vi "Drive Controller.vi"(8 "error in":errorcluster) -> ()   [LabVIEW 2020]
doc: "This VI executes continuously carrying out the current operation and responding to updates or new operation requests. It will often contain the timing or control code that is difficult to place directly in TeleOp. This VI generally opens all sensors and motors and isolates the rest of the robot code from knowing implementation details of how the operations are carried out."
uses:
  <vilib>/Rock Robotics/WPI/Framework/Completion Status.ctl
  Drive Setpoints.ctl
  Drive Operations.ctl
  <vilib>/Rock Robotics/WPI/SafetyOutput/WPI_SafetyOutputConfigMenu.ctl
  <vilib>/Rock Robotics/WPI/RobotDrive/WPI_RobotDriveOpen2MotorWithExistingMotors.vi
  <vilib>/Rock Robotics/Network Tables/NT Write Numeric Array.vi
panel:
  in  "Interactive Values":T1
  in  "Buttons":cluster{"Execute Cmd":bool, "Abort Cmd":bool}
  out "Command Timing":cluster{"Start Time (ms)":u32, "Iterations":i32}
  out "Status":T3
  out "Setpoints":T4(graph)
  out "Current\nCmd":string
  # "Tip: The graph shows the motor setpoints. It may also be helpful to observe inputs and sensor values.\nYou may also want to display tuning or debugging controls."
  # "Interactive Command: You may fill in the settings for a command\nand schedule it with the Execute button. You can observe and abort\nany command while fine tuning the code for the controller."
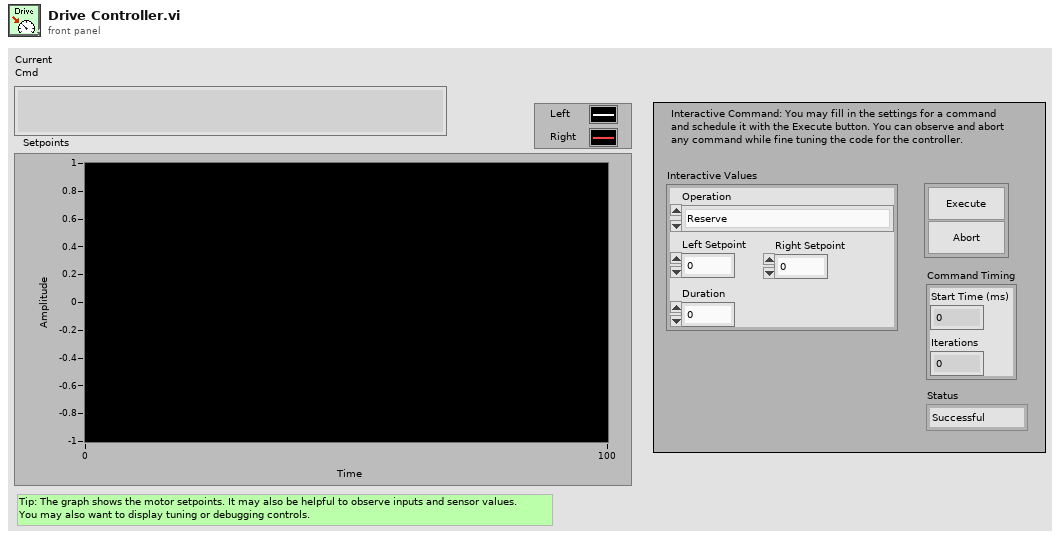
[diagram p1: front panel]
types:
  T1 = typedef "Drive Setpoints.ctl" = cluster{"Operation":T2, "Left Setpoint":dbl, "Right Setpoint":dbl, "Duration":dbl}
  T2 = typedef "Drive Operations.ctl" = enum16{"Reserve", "Read Current", "Immediate", "Drive for Time", "Drive for Distance"}
  T3 = typedef "Completion Status.ctl" = enum16{"Successful", "Aborted", "Incomplete"}
  T4 = cluster{"Left Setpoint":dbl, "Right Setpoint":dbl}
  T5 = typedef "WPI_SafetyOutputConfigMenu.ctl" = enum16{"Enable", "Disable"}
  T6 = typedef "WPI_MotorControlDeviceRef.ctl" = cluster{"DeviceStatus":errorcluster, "Type":T7, "PWM":cluster{"PWM Channel":T8, "DeadBand":T9}, "CAN":cluster{"Device Number":u8, "SetOutput VI Ref":variant, "GetOutput VI Ref":variant, "Enable VI Ref":variant, "Disable VI Ref":variant, "Data":variant}, "Invert":bool, "DIO PWM":cluster{"PWM \"Enable\" Channel":T8, "DIOChannel":T10, "PWM Rate":dbl}}
  T7 = typedef "WPI_MotorControlType.ctl" = enum16{"PWM", "CAN", "DIO PWM"}
  T8 = typedef "FPGA_DIOPWMChannel.ctl" = enum8{"PWM 0", "PWM 1", "PWM 2", "PWM 3", "PWM 4", "PWM 5", "PWM 6", "PWM 7", "PWM 8", "PWM 9", "PWM MXP 0", "PWM MXP 1", "PWM MXP 2", "PWM MXP 3", "PWM MXP 4", "PWM MXP 5", "PWM MXP 6", "PWM MXP 7", "PWM MXP 8", "PWM MXP 9", "Invalid"}
  T9 = typedef "WPI_PWMDeadband.ctl" = cluster{"Name":string, "maxPositivePwm":i32, "minPositivePwm":i32, "centerPwm":i32, "maxNegativePwm":i32, "minNegativePwm":i32, "angularRange":u16}
  T10 = typedef "FPGA_DIOChannel.ctl" = enum8{"DIO 0", "DIO 1", "DIO 2", "DIO 3", "DIO 4", "DIO 5", "DIO 6", "DIO 7", "DIO 8", "DIO 9", "DIO MXP 0", "DIO MXP 1", "DIO MXP 2", "DIO MXP 3", "DIO MXP 4", "DIO MXP 5", "DIO MXP 6", "DIO MXP 7", "DIO MXP 8", "DIO MXP 9", "DIO MXP 10", "DIO MXP 11", "DIO MXP 12", "DIO MXP 13", "DIO MXP 14", "DIO MXP 15", "SPI Port CS1", "SPI Port CS2", "SPI Port CS3", "SPI Port MISO", "SPI Port MOSI", "Invalid"}
  T11 = typedef "WPI_RobotDriveDevRef.ctl" = cluster{"DevStatus":errorcluster, "Motors[]":T6[], "Square Inputs":bool, "Max Output":dbl}
  T12 = typedef "Command Status Info.ctl" = cluster{"Name":string, "Status":T3, "notifier out":T13}
  T13 = typedef "Completion Notifier.ctl" = refnum<notifier>
  T14 = cluster{"SubSystem Data":T1, cluster{"Start Time (ms)":u32, "Iterations":i32}, cluster{"Command Info":T12, "Description":string, "Default Command":T1, "queue out":refnum<queue>, "Subsystem Name":string}}
  T15 = cluster{"SubSystem Data":T1, cluster{"Start Time (ms)":u32, "Iterations":i32}, "Default Command Arguments":cluster{"Command Info":T12, "Description":string, "Default Command":T1, "queue out":refnum<queue>, "Subsystem Name":string}}
  T16 = cluster{"Don't move motors while reserved":dbl, "Don't move motors while reserved":dbl}
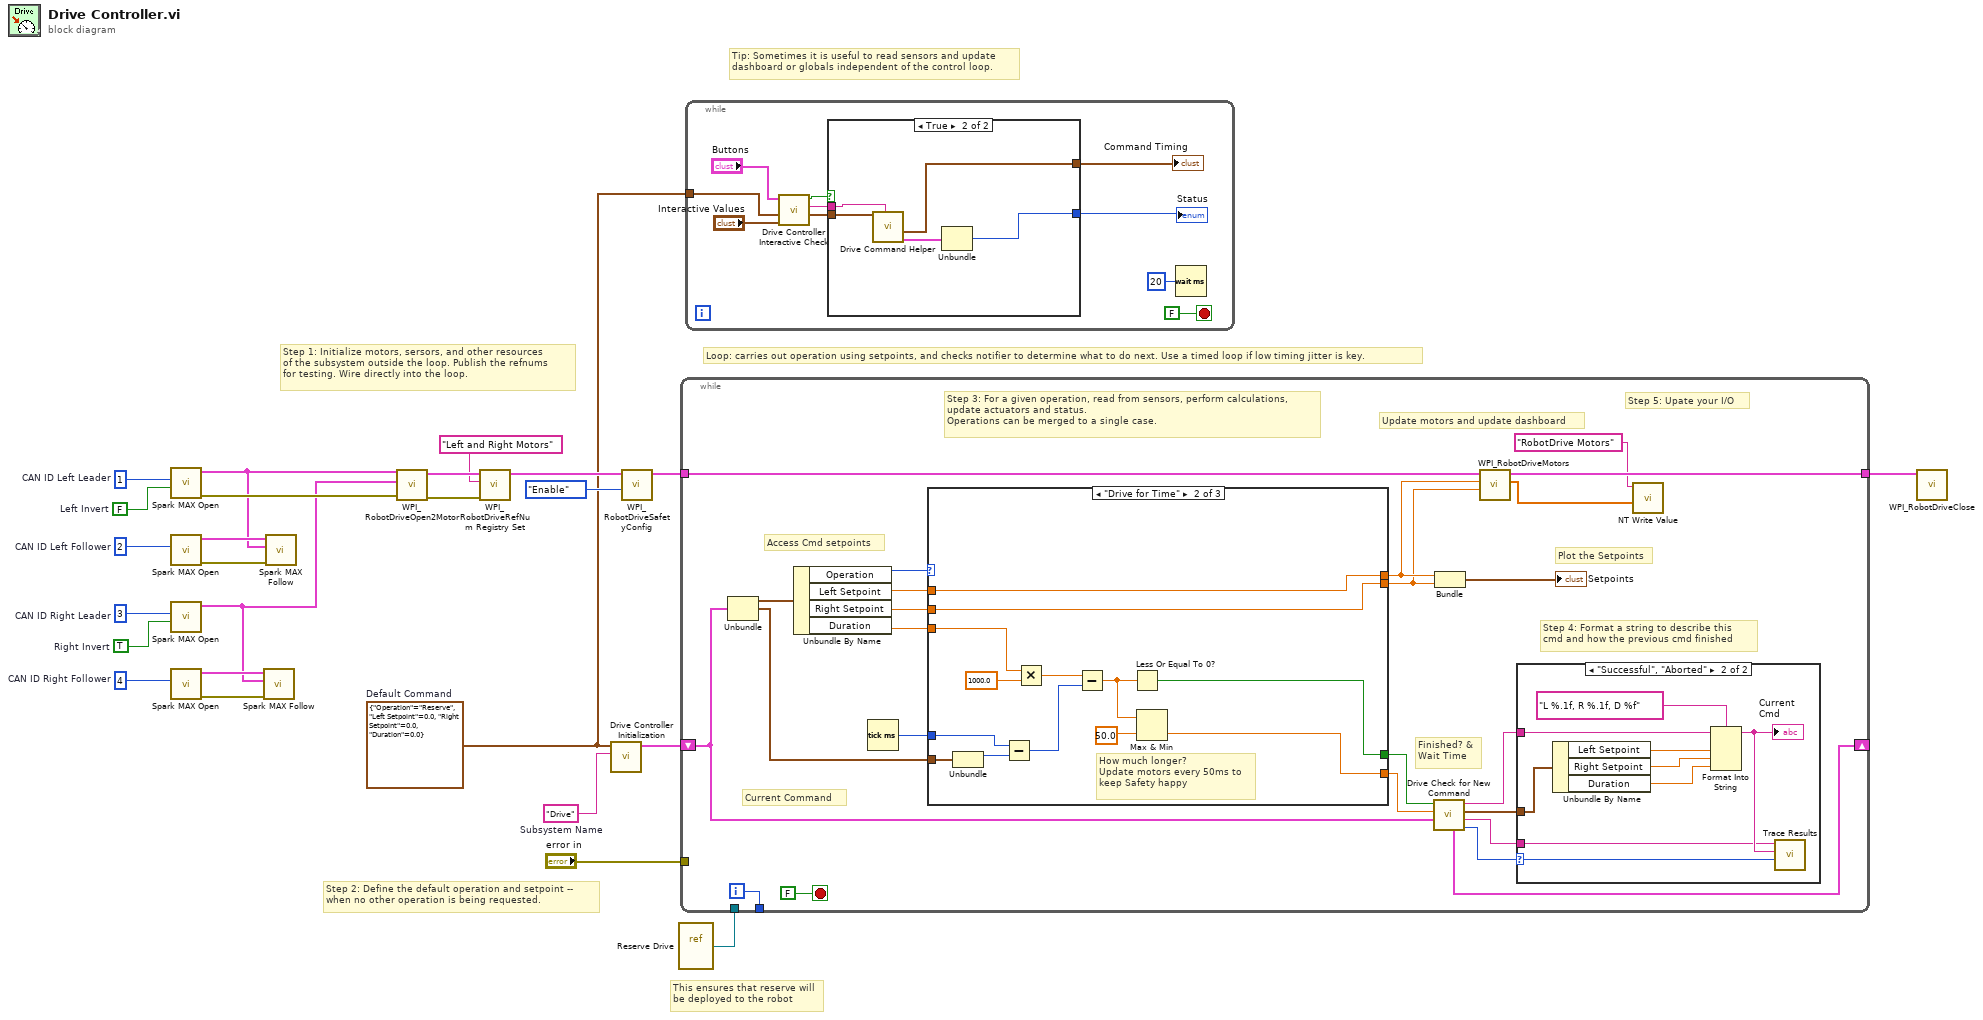
[diagram p0: block diagram]
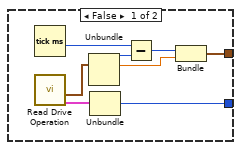
[diagram p2: hidden frame]
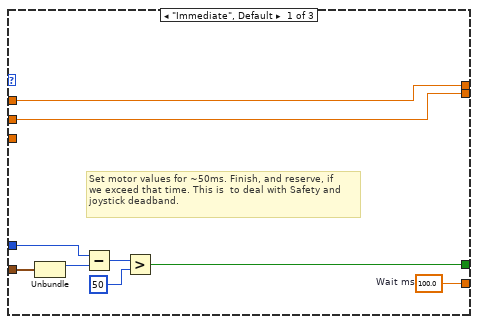
[diagram p4: hidden frame]
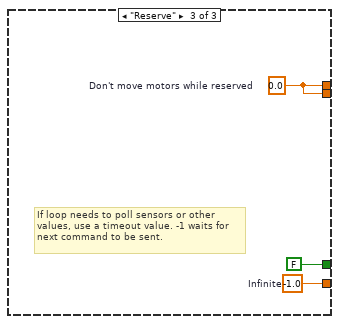
[diagram p5: hidden frame]
diagram:
  w2 = TRUE  # Right Invert
  w3 = FALSE  # Left Invert
  w4 = u8 4  # CAN ID Right Follower
  w5 = u8 3  # CAN ID Right Leader
  w6 = u8 2  # CAN ID Left Follower
  w7 = u8 1  # CAN ID Left Leader
  w15 = T1 {"Operation"=enum."Reserve", "Left Setpoint"=0.0, "Right Setpoint"=0.0, "Duration"=0.0}  # Default Command
  w25 = "Drive"  # Subsystem Name
  # "This ensures that reserve will\nbe deployed to the robot"
  # "Tip: Sometimes it is useful to read sensors and update\ndashboard or globals independent of the control loop."
  # "Step 2: Define the default operation and setpoint --\nwhen no other operation is being requested."
  # "Step 1: Initialize motors, sersors, and other resources\nof the subsystem outside the loop. Publish the refnums\nfor testing. Wire directly into the loop."
  # "Loop: carries out operation using setpoints, and checks notifier to determine what to do next. Use a timed loop if low timing jitter is key."
  n1 = call <vilib>:"Spark MAX Open.vi"("Invert"=w3, "Device Number"=w7) -> ("error out"=w14:errorcluster, "MotorControlDeviceRef"=w9:T6)  [unwired: 8 in]
  n2 = call <vilib>:"Spark MAX Open.vi"("Device Number"=w6) -> ("error out"=w12:errorcluster, "MotorControlDeviceRef"=w13:T6)  [unwired: 9 in]
  n3 = call <vilib>:"Spark MAX Open.vi"("Invert"=w2, "Device Number"=w5) -> ("MotorControlDeviceRef"=w8:T6)  [unwired: 8 in, 1 out]
  n4 = call <vilib>:"Spark MAX Open.vi"("Device Number"=w4) -> ("error out"=w10:errorcluster, "MotorControlDeviceRef"=w11:T6)  [unwired: 9 in]
  n5 = call <vilib>:"Spark MAX Follow.vi"("error in (no error)"=w10, "Master Controller"=w8, "MotorControlDeviceRef"=w11) -> ()  [unwired: 7 in, 2 out]
  n6 = call <vilib>:"Spark MAX Follow.vi"("error in (no error)"=w12, "Master Controller"=w9, "MotorControlDeviceRef"=w13) -> ()  [unwired: 7 in, 2 out]
  n7 = call-poly <vilib>:"WPI_RobotDriveOpen2Motor.vi"("error in (no error)"=w14, "Right Motor Dev Ref"=w8, "Left Motor Dev Ref"=w9) -> ("error out"=w22:errorcluster, "RobotDriveDevRef"=w24:T11)  [unwired: 2 in, 5 out]
  n8 = call <vilib>:"WPI_RobotDriveRefNum Registry Set.vi"("error in (no error)"=w22, "refnum name"="Left and Right Motors", "RobotDriveDevRef"=w24) -> ("RobotDriveDevRef"=w21:T11)  [unwired: 1 in, 7 out]
  n9 = call "Drive Controller Initialization.vi"("Subsystem Name"=w25, "Default Command"=w15) -> ("Current Command"=w17:T14)  [unwired: 9 in]
  n10 = call <vilib>:"WPI_RobotDriveSafetyConfig.vi"("mode"=WPI_SafetyOutputConfigMenu."Enable", "RobotDriveDevRef"=w21) -> ("RobotDriveDevRef"=w19:T11)  [unwired: 8 in, 1 out]
  n11 = vi-ref "Reserve Drive.vi"() -> (w16:refnum<vi>)
  n12 = while {
    shift-right: [w36] -> _
    shift-left: w17 -> [w29]
    tunnel: [w48] -> _
    tunnel: w19 -> [w44]
    tunnel: "error in" -> [_]
    tunnel: w16 -> [_]
    tunnel: [w28] -> w1
    i -> [w48]
    stop <- FALSE stop-if-true
    # "Step 5: Upate your I/O"
    # "Step 4: Format a string to describe this\ncmd and how the previous cmd finished"
    # "Current Command"
    # "Update motors and update dashboard"
    # "Plot the Setpoints"
    # "Access Cmd setpoints"
    # "Finished? &\nWait Time"
    # "Step 3: For a given operation, read from sensors, perform calculations,\nupdate actuators and status.\nOperations can be merged to a single case."
    n13 = Unbundle(w29) -> ("SubSystem Data"=w43:T1, w30:cluster{"Start Time (ms)":u32, "Iterations":i32})  [unwired: 1 out]
    n14 = Unbundle By Name(w43) -> ("Operation"=w42:T2, "Left Setpoint"=w41:dbl, "Right Setpoint"=w40:dbl, "Duration"=w39:dbl)
    n15 = Tick Count (ms)() -> (millisecond timer value=w38:u32)
    n16 = case shown="\"Drive for Time\"" w42 {
      tunnel: [w67 w68 w83] -> w35
      tunnel: [w60 w75 FALSE ("ignore previous (F)")] -> w34
      tunnel: w30 -> [w59 w77 _]
      tunnel: [w66 w74 w81] -> w46
      tunnel: [w65 w73 w81] -> w45
      tunnel: w41 -> [w66 w74 _]
      tunnel: w40 -> [w65 w73 _]
      tunnel: w39 -> [_ w72 _]
      tunnel: w38 -> [w61 w71 _]
      frame "Immediate", Default {
        w67 = 100.0  # Wait ms
        # "Set motor values for ~50ms. Finish, and reserve, if\nwe exceed that time. This is  to deal with Safety and\njoystick deadband."
        n17 = Unbundle(w59) -> ("Start Time (ms)"=w62:u32)  [unwired: 1 out]
        n18 = Subtract(x=w61, y=w62) -> (x-y=w63:u32)
        n19 = Greater?(x=w63, y=u8 50 ("Left Motor")) -> (0:w60:bool)
      }
      frame "Drive for Time" {
        # "How much longer?\nUpdate motors every 50ms to\nkeep Safety happy"
        n20 = Unbundle(w77) -> ("Start Time (ms)"=w76:u32)  [unwired: 1 out]
        n21 = Subtract(x=w71, y=w76) -> (x-y=w80:u32)
        n22 = Multiply(x=w72, y=1000.0) -> (x*y=w79:dbl)
        n23 = Subtract(x=w79, y=w80) -> (x-y=w70:dbl)
        n24 = Less Or Equal To 0?(x=w70) -> (x <= 0?=w75:bool)
        n25 = Max & Min(x=w70, y=50.0) -> (min(x,y)=w68:dbl)  [unwired: 1 out]
      }
      frame "Reserve" {
        w81 = 0.0  # Don't move motors while reserved
        w83 = -1.0  # Infinite
        # "If loop needs to poll sensors or other\nvalues, use a timeout value. -1 waits for\nnext command to be sent."
      }
    }
    n26 = call "Drive Check for New Command.vi"("input cluster"=w29, "Wait time (ms)"=w35, "Finished?"=w34) -> ("Completion"=w37:T3, "Subsystem Name"=w31:string, "Current Command"=w32:T1, "Initial Trace String"=w33:string, "Next Command"=w36:T15)  [unwired: 4 in]
    n27 = Bundle("Don't move motors while reserved"=w46, "Don't move motors while reserved"=w45) -> (→"Setpoints":T16)  [unwired: 1 in]
    n28 = call <vilib>:"WPI_RobotDriveMotors.vi"("RightSpeed"=w45, "LeftSpeed"=w46, "RobotDriveDevRef"=w44) -> ("Motor Values"=w27:dbl[], "RobotDriveDevRef"=w28:T11)  [unwired: 1 in, 6 out]
    n29 = case shown="\"Successful\", \"Aborted\"" w37 {
      selector: w37 -> [_ w58]
      tunnel: w33 -> [_ w53]
      tunnel: w32 -> [_ w54]
      tunnel: w31 -> [_ w50]
      frame "Incomplete", Default {
        # "Continuing current command"
      }
      frame "Successful", "Aborted" {
        # "Report and setup for next command"
        n30 = Unbundle By Name(w54) -> ("Left Setpoint"=w56:dbl, "Right Setpoint"=w57:dbl, "Duration"=w51:dbl)
        n31 = Format Into String(format string="L %.1f, R %.1f, D %f", initial string=w53, w56, w57, w51) -> (resulting string=w52:string)  [unwired: 1 in, 1 out]
        "Current\nCmd" <- w52
        n32 = call <vilib>:"Trace Results.vi"("Status of previous command"=w58, "Description"=w52, "Subsystem"=w50) -> ()  [unwired: 9 in]
      }
    }
    n33 = call-poly <vilib>:"NT Write Value.vi"("Numeric Array"=w27, "Name"="RobotDrive Motors") -> ()  [unwired: 9 in, 1 out]
  }
  n34 = while {
    tunnel: w15 -> [w85]
    stop <- FALSE stop-if-true
    n35 = call "Drive Controller Interactive Check.vi"("Interactive Command In"="Interactive Values", "Default Command"=w85, "Buttons"="Buttons") -> ("Interactive Command Out"=w87:T1, "Trace String"=w88:string, "Schedule"=w89:bool)  [unwired: 6 in]
    n36 = case shown="True" w89 {
      tunnel: [w98 w106] -> w90
      tunnel: [w97 w102] -> w91
      tunnel: w88 -> [_ w104]
      tunnel: w87 -> [_ w103]
      frame False {
        n37 = Tick Count (ms)() -> (millisecond timer value=w101:u32)
        n38 = call "Read Drive Operation.vi"() -> ("Command Info"=w95:T12, "SubSystem Data"=w94:T1)  [unwired: 9 in, 1 out]
        n39 = Unbundle(w94) -> ("Operation"=w99:T2, "Left Setpoint"=w96:dbl)  [unwired: 2 out]
        n40 = Unbundle(w95) -> ("Status"=w98:T3)  [unwired: 2 out]
        n41 = Subtract(x=w101, y=w99) -> (x-y=w100:u32)
        n42 = Bundle(w100, "Left Setpoint"=w96) -> (w97:cluster{u32, "Left Setpoint":dbl})  [unwired: 1 in]
      }
      frame True {
        n43 = call "Drive Command Helper.vi"("Description"=w104, "SubSystem Data"=w103) -> ("Command Info Out"=w105:T12, "Command Timing"=w102:cluster{"Start Time (ms)":u32, "Iterations":i32})  [unwired: 7 in, 1 out]
        n44 = Unbundle(w105) -> ("Status"=w106:T3)  [unwired: 2 out]
      }
    }
    "Status" <- w90
    "Command Timing" <- w91
    n45 = Wait (ms)(milliseconds to wait=u32 20) -> ()  [unwired: 1 out]
  }
  n46 = call <vilib>:"WPI_RobotDriveClose.vi"("RobotDriveDevRef"=w1) -> ()  [unwired: 10 in, 1 out]
